vi "CompareAnkleSpeed.vi"(4 "Init (F)":bool, 6 "Direction":T2, 8 "dt":dbl=0.01, 9 "Minimum Speed":dbl=0.4 format="%#_13g", 10 "AnkleInGCS":dbl[](array[numeric]), 11 "GaitPhase":T1) -> (0 "Filtered Ankle Speed":dbl[](array[numeric]), 3 "Ankle Speed Changed":bool)   [LabVIEW 2016, in "ForceField.lvclass"]
uses:
  ForceField.lvclass
  SerialChain/TypeDef/xyzO.ctl
  TypeDef/GaitPhase.ctl
  <vilib>/ptbypt/NI_PtbyPt.lvlib
  SerialChain/SerialChain.lvclass
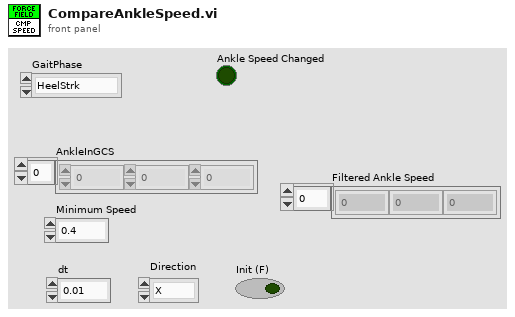
[diagram p1: front panel]
types:
  T1 = typedef "ForceField.lvclass/GaitPhase.ctl" = enum16{"HeelStrk", "Stance", "ToeOff", "Swing"}
  T2 = typedef "SerialChain.lvclass/xyzO.ctl" = enum16{"X", "Y", "Z", "O"}
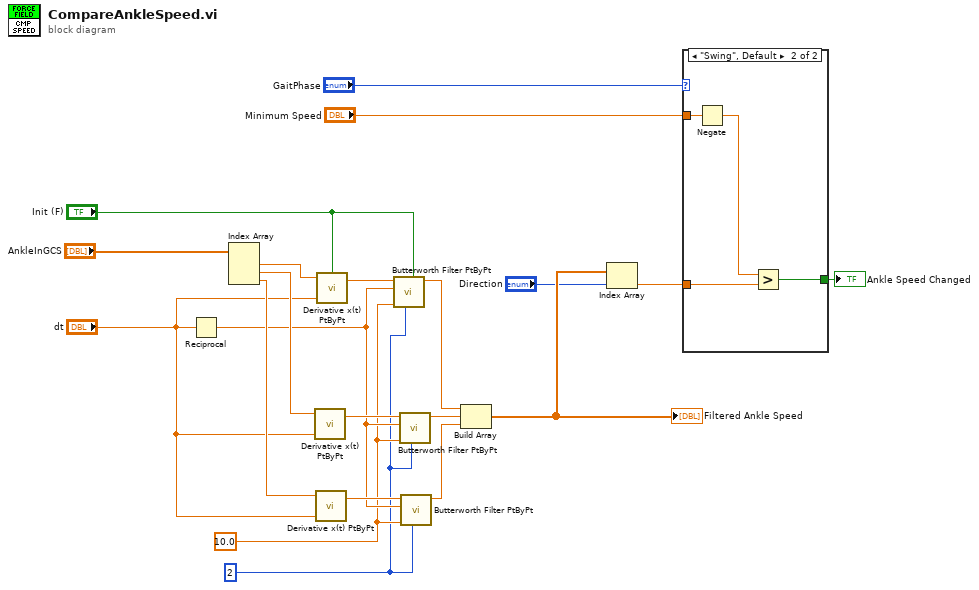
[diagram p0: block diagram]
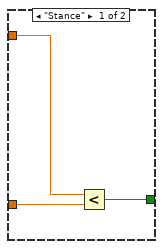
[diagram p2: hidden frame]
diagram:
  w8 = 10.0 ("low cutoff freq: fl")
  w7 = 2 ("order")
  n1 = Reciprocal(x="dt") -> (1/x=w9:dbl)
  n2 = Index Array(array="AnkleInGCS") -> (element #1=w19:dbl, element #2=w12:dbl, element #3=w11:dbl)  [unwired: 3 in]
  n3 = call <vilib>:"Derivative x(t) PtByPt.vi"("dt"="dt", "x"=w12) -> ("dx/dt"=w14:dbl)  [unwired: 2 in, 1 out]
  n4 = call <vilib>:"Derivative x(t) PtByPt.vi"("dt"="dt", "x"=w11) -> ("dx/dt"=w13:dbl)  [unwired: 2 in, 1 out]
  n5 = call <vilib>:"Derivative x(t) PtByPt.vi"("initialize"="Init (F)", "dt"="dt", "x"=w19) -> ("dx/dt"=w18:dbl)  [unwired: 1 in, 1 out]
  n6 = call <vilib>:"Butterworth Filter PtByPt.vi"("initialize"="Init (F)", "order"=w7, "low cutoff freq: fl"=w8, "sampling freq: fs"=w9, "x"=w18) -> ("Filtered x"=w4:dbl)  [unwired: 4 in, 1 out]
  n7 = call <vilib>:"Butterworth Filter PtByPt.vi"("order"=w7, "low cutoff freq: fl"=w8, "sampling freq: fs"=w9, "x"=w14) -> ("Filtered x"=w5:dbl)  [unwired: 5 in, 1 out]
  n8 = call <vilib>:"Butterworth Filter PtByPt.vi"("order"=w7, "low cutoff freq: fl"=w8, "sampling freq: fs"=w9, "x"=w13) -> ("Filtered x"=w6:dbl)  [unwired: 5 in, 1 out]
  n9 = Build Array(w4, w5, w6) -> (w3:dbl[])
  "Filtered Ankle Speed" <- w3
  n10 = Index Array(array=w3, index="Direction") -> (element=w1:dbl)
  n11 = case shown="\"Swing\", Default" "GaitPhase" {
    tunnel: w1 -> [w23 w27]
    tunnel: "Minimum Speed" -> [w24 w28]
    tunnel: [w22 w26] -> w15
    frame "Stance" {
      n12 = Less?(x=w24, y=w23) -> (x < y?=w22:bool)
    }
    frame "Swing", Default {
      n13 = Negate(x=w28) -> (-x=w25:dbl)
      n14 = Greater?(x=w25, y=w27) -> (0:w26:bool)
    }
  }
  "Ankle Speed Changed" <- w15
